vi "Interface.Error Queue.Write.vi"(7 "FIFO Debug Flags":refnum<class "FIFO Flags.lvclass">, 8 "error in (no error)":errorcluster, 9 "timeout in ms (0)":i32 format="%d ms", 10 "element":errorcluster, 11 "Error Queue in":T1) -> (0 "error out":errorcluster, 1 "timed out?":bool, 3 "Error Queue out":T1)   [LabVIEW 2017, in "DSF Core.lvlib" / "Interface.lvclass"]
uses:
  Interface.lvclass
  Interface.Error Queue.Ref.ctl
  Debug/FIFO Flags.lvclass
  Debug/FIFO Flags.lvclass/FIFO Flags.ctl
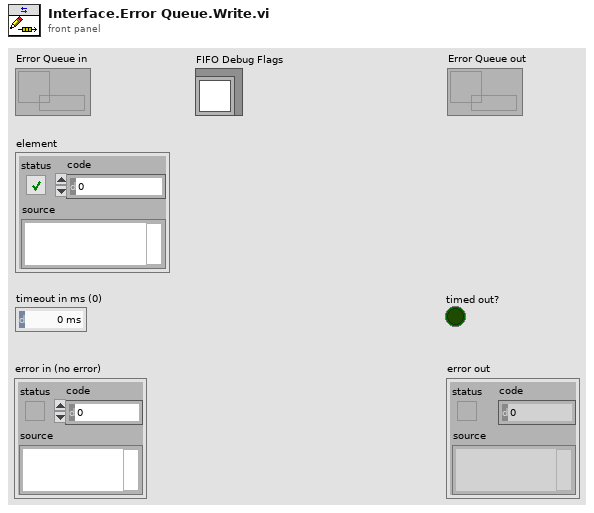
[diagram p1: front panel]
types:
  T1 = typedef "DSF Core.lvlib/Interface.lvclass/Interface.Error Queue.Ref.ctl" = refnum<queue>
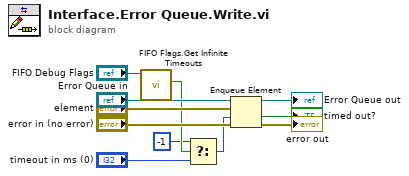
[diagram p0: block diagram]
diagram:
  n1 = call "FIFO Flags.Get Infinite Timeouts.vi"("FIFO Debug Flags in"="FIFO Debug Flags") -> ("infinite timeouts"=w5:bool)  [unwired: 9 in, 1 out]
  n2 = Select(t=-1, s=w5, f="timeout in ms (0)") -> (s? t:f=w2:i32)
  n3 = Enqueue Element(queue="Error Queue in", element="element", timeout in ms (-1)=w2, error in (no error)="error in (no error)") -> (queue out=→"Error Queue out":T1, timed out?=→"timed out?":bool, error out=→"error out":errorcluster)
